vi "threshold fraction or count.vi"(10 "Threshold in":dbl, 11 "Maximal Value":sgl) -> (3 "Threshold out":dbl)   [LabVIEW 2013]
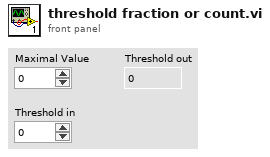
[diagram p1: front panel]
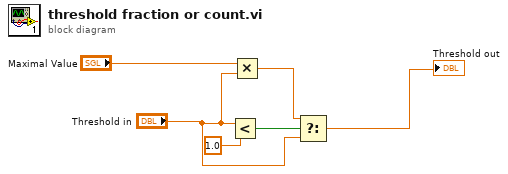
[diagram p0: block diagram]
diagram:
  n1 = Less?(x="Threshold in", y=1.0) -> (x < y?=w3:bool)
  n2 = Multiply(x="Maximal Value", y="Threshold in") -> (x*y=w4:dbl)
  n3 = Select(t=w4, s=w3, f="Threshold in") -> (s? t:f=→"Threshold out":dbl)
